vi "Source tag - defaulting.vi"(8 "error in (no error)":errorcluster) -> (0 "error out":errorcluster)   [LabVIEW 2026, in "Tests.lvlib"]
doc: "Unit test (Caraya) for source-tag defaulting and sanitization.\nVerifies that when a caller supplies no tag, the tag defaults to the origin VI's base name with the .vi extension stripped and any remaining dots replaced by underscores, so a VI filename containing dots cannot be misread as tag hierarchy (the default is always a single node). Also verifies Sanitize directly and that an explicitly supplied tag is preserved verbatim.\nPure test: no actors, no file I/O, no fixture. Reaches the protected Tag helpers via the Tests.lvlib friend relationship.\n\nImplements LMBR-T-017, T-018, T-019 -> SRS-013, SRS-017. Assert-level IDs: Test-ID-Assert-Checklist.md."
uses:
  Tests.lvlib
  <vilib>/addons/_JKI Toolkits/Caraya/classes/Assert/Assert Equal Value_Variant.vi
  <vilib>/addons/_JKI Toolkits/Caraya/classes/Test/Test.lvclass
  <vilib>/addons/_JKI Toolkits/Caraya/classes/Assert/Assert.lvclass
  src/Lumberjack.lvlib
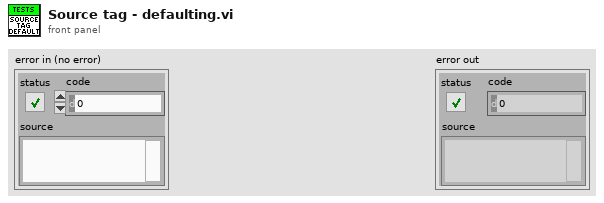
[diagram p1: front panel]
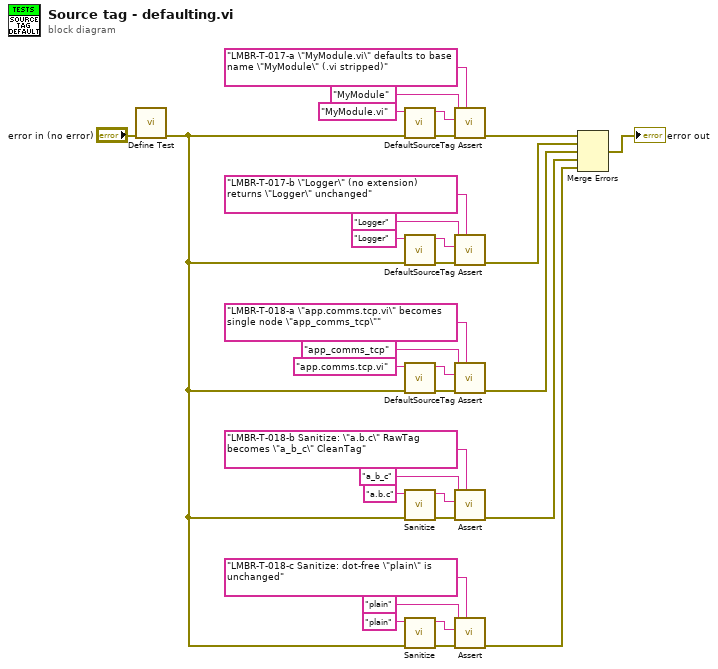
[diagram p0: block diagram]
diagram:
  n1 = call <vilib>:"Define Test.vi"("error in (no error)"="error in (no error)") -> ("error out"=w5:errorcluster)  [unwired: 9 in, 1 out]
  n2 = call "DefaultSourceTag.vi"("error in (no error)"=w5, "OriginVI"="MyModule.vi") -> ("error out"=w31:errorcluster, "SourceTag"=w30:string)  [unwired: 8 in]
  n3 = call "DefaultSourceTag.vi"("error in (no error)"=w5, "OriginVI"="Logger") -> ("error out"=w25:errorcluster, "SourceTag"=w24:string)  [unwired: 8 in]
  n4 = call "DefaultSourceTag.vi"("error in (no error)"=w5, "OriginVI"="app.comms.tcp.vi") -> ("error out"=w20:errorcluster, "SourceTag"=w19:string)  [unwired: 8 in]
  n5 = call "Sanitize.vi"("error in (no error)"=w5, "RawTag"="a.b.c" ("OriginVI")) -> ("error out"=w15:errorcluster, "CleanTag"=w14:string)  [unwired: 8 in]
  n6 = call "Sanitize.vi"("error in (no error)"=w5, "RawTag"="plain" ("OriginVI")) -> ("error out"=w10:errorcluster, "CleanTag"=w9:string)  [unwired: 8 in]
  n7 = call-poly <vilib>:"Assert.vi"("Label"="LMBR-T-017-a \"MyModule.vi\" defaults to base name \"MyModule\" (.vi stripped)", "error in (no error)"=w31, "Actual"=w30, "Expected"="MyModule" ("OriginVI")) -> ("error out"=w26:errorcluster)  [unwired: 6 in, 1 out]
  n8 = call-poly <vilib>:"Assert.vi"("Label"="LMBR-T-017-b \"Logger\" (no extension) returns \"Logger\" unchanged", "error in (no error)"=w25, "Actual"=w24, "Expected"="Logger" ("OriginVI")) -> ("error out"=w4:errorcluster)  [unwired: 6 in, 1 out]
  n9 = call-poly <vilib>:"Assert.vi"("Label"="LMBR-T-018-a \"app.comms.tcp.vi\" becomes single node \"app_comms_tcp\"", "error in (no error)"=w20, "Actual"=w19, "Expected"="app_comms_tcp" ("OriginVI")) -> ("error out"=w3:errorcluster)  [unwired: 6 in, 1 out]
  n10 = call-poly <vilib>:"Assert.vi"("Label"="LMBR-T-018-b Sanitize: \"a.b.c\" RawTag becomes \"a_b_c\" CleanTag", "error in (no error)"=w15, "Actual"=w14, "Expected"="a_b_c" ("OriginVI")) -> ("error out"=w2:errorcluster)  [unwired: 6 in, 1 out]
  n11 = call-poly <vilib>:"Assert.vi"("Label"="LMBR-T-018-c Sanitize: dot-free \"plain\" is unchanged", "error in (no error)"=w10, "Actual"=w9, "Expected"="plain" ("OriginVI")) -> ("error out"=w1:errorcluster)  [unwired: 6 in, 1 out]
  n12 = Merge Errors(w26, w4, w3, w2, w1) -> (→"error out":errorcluster)
